vi "main.vi"   [LabVIEW 2015]
uses:
  <vilib>/addons/Modulation/niDMT.lvlib
  <vilib>/addons/Modulation/niAMT.lvlib
  <vilib>/addons/Modulation/Digital/General/MT Format Eye Diagram (complex).vi
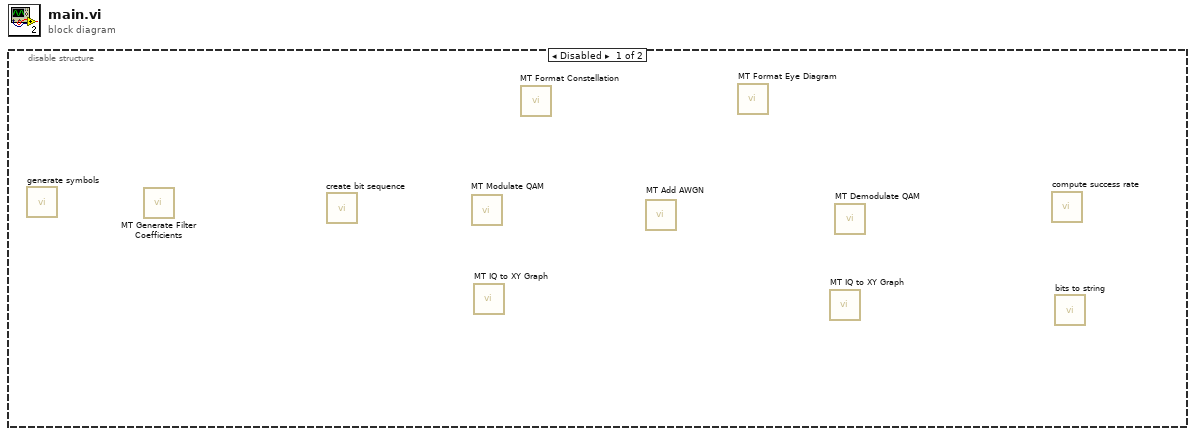
[diagram p0: block diagram]
diagram:
  n1 = disable-structure shown="Disabled" {
    frame Disabled {
      n2 = call "generate symbols.vi"() -> ()  [unwired: 11 in, 1 out]
      n3 = call <vilib>:"MT Generate Filter Coefficients.vi"() -> ()  [unwired: 13 in, 3 out]
      n4 = call "create bit sequence.vi"() -> ()  [unwired: 10 in, 2 out]
      n5 = call <vilib>:"MT Modulate QAM.vi"() -> ()  [unwired: 13 in, 3 out]
      n6 = call <vilib>:"MT IQ to XY Graph.vi"() -> ()  [unwired: 13 in, 3 out]
      n7 = call <vilib>:"MT Format Constellation.vi"() -> ()  [unwired: 14 in, 2 out]
      n8 = call <vilib>:"MT Add AWGN.vi"() -> ()  [unwired: 13 in, 3 out]
      n9 = call-poly <vilib>:"MT Format Eye Diagram.vi"() -> ()  [unwired: 14 in, 2 out]
      n10 = call <vilib>:"MT IQ to XY Graph.vi"() -> ()  [unwired: 13 in, 3 out]
      n11 = call <vilib>:"MT Demodulate QAM.vi"() -> ()  [unwired: 11 in, 5 out]
      n12 = call "compute success rate.vi"() -> ()  [unwired: 11 in, 1 out]
      n13 = call "bits to string.vi"() -> ()  [unwired: 11 in, 1 out]
    }
    frame Enabled {
    }
  }
